vi "Test XYZ Output Channel List.vi"() -> (0 "Reason":string, 1 "Success":bool)   [LabVIEW 2013]
uses:
  <vilib>/xml/Load XML File.vi
  <vilib>/xml/NI_XML.lvlib
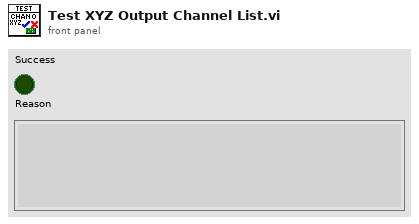
[diagram p1: front panel]
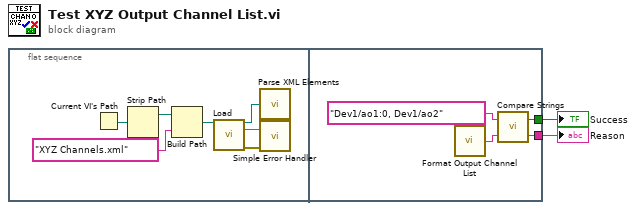
[diagram p0: block diagram]
diagram:
  n1 = flat-sequence {
    tunnel: [w11] -> w2
    tunnel: [w10] -> w1
    frame #0 {
      n2 = Current VI's Path() -> (path=w9:path)
      n3 = Strip Path(path=w9) -> (stripped path=w8:path)  [unwired: 1 out]
      n4 = Build Path(base path=w8, name or relative path="XYZ Channels.xml") -> (appended path=w3:path)
      n5 = call-poly <vilib>:"Load.vi"("path to XML document"=w3) -> ("DOM document out"=w6:refnum<k20>, "parse errors"=w4:string, "error out"=w5:errorcluster)  [unwired: 12 in]
      n6 = call "Parse XML Elements.vi"("DOM"=w6) -> ()
      n7 = call <vilib>:"Simple Error Handler.vi"("error source (\" \")"=w4, "error in (no error)"=w5) -> ()  [unwired: 3 in, 5 out]
    }
    frame #1 {
      n8 = call "Format Output Channel List.vi"() -> ("Output Channels"=w12:string)
      n9 = call "Compare Strings.vi"("Got"=w12, "Wanted"="Dev1/ao1:0, Dev1/ao2" ("Input Channels")) -> ("Reason"=w10:string, "Success"=w11:bool)
    }
  }
  "Success" <- w2
  "Reason" <- w1
